vi "Rename and Replace Module Class.vi"(8 "error in (no error)":errorcluster, 10 "New Module/Lib Name":string, 11 "ProjectItem in":refnum<vi>) -> (0 "error out":errorcluster)   [LabVIEW 2015, in "Generic Module Library.lvlib"]
uses:
  Generic Module Library.lvlib
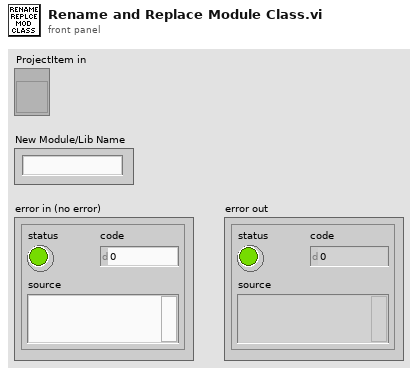
[diagram p1: front panel]
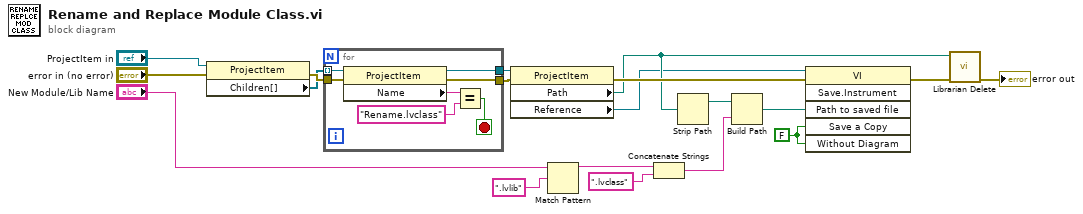
[diagram p0: block diagram]
diagram:
  w5 = FALSE ("Save a Copy")
  n1 = property on="Property Node" class="ProjectItem"(reference="ProjectItem in", error in="error in (no error)") -> (error out=w19:errorcluster, "Children[]"=w3:refnum<vi>[])  [unwired: 1 out]
  n2 = for {
    tunnel: w3 -> [w26] mode=indexing
    tunnel: [w22] -> w4
    tunnel: [w21] -> w18
    tunnel: w19 -> [w20]
    stop <- w23 stop-if-true
    n3 = property class="ProjectItem"(reference=w26, error in=w20) -> (reference out=w22:refnum<vi>, error out=w21:errorcluster, "Name"=w25:string)
    n4 = Equal?(x=w25, y="Rename.lvclass") -> (x = y?=w23:bool)
  }
  n5 = property class="ProjectItem"(reference=w4, error in=w18) -> (error out=w17:errorcluster, "Path"=w8:path, "Reference"=w7:refnum<vi>)  [unwired: 1 out]
  n6 = Match Pattern(string="New Module/Lib Name", regular expression=".lvlib") -> (before substring=w14:string)  [unwired: 1 in, 3 out]
  n7 = Concatenate Strings(w14, ".lvclass" ("string")) -> (w10:string)
  n8 = Strip Path(path=w8) -> (stripped path=w9:path)  [unwired: 1 out]
  n9 = Build Path(base path=w9, name or relative path=w10) -> (appended path=w12:path)
  n10 = invoke class="VI" method="Save.Instrument"(reference=w7, error in=w17, "Path to saved file"=w12, "Save a Copy"=w5, "Without Diagram"=w5) -> (error out=w6:errorcluster)  [unwired: 1 in, 5 out]
  n11 = call <vilib>:"Librarian Delete.vi"("error in (no error)"=w6, "path"=w8) -> ("error out"=→"error out":errorcluster)  [unwired: 9 in]
